vi "DSF.Engine.Interface.RT FIFO.Create.vi"(7 "size (10)":u32, 8 "error in (no error)":errorcluster) -> (0 "error out":errorcluster, 3 "RT FIFO":T1)   [LabVIEW 2016, in "DSF.Engine.lvlib" / "DSF.Engine.Interface.lvclass"]
uses:
  DSF.Engine.Interface.lvclass
  DSF.Engine.Interface.RT FIFO Ref.ctl
  DSF.Engine.Interface.RT FIFO Data.ctl
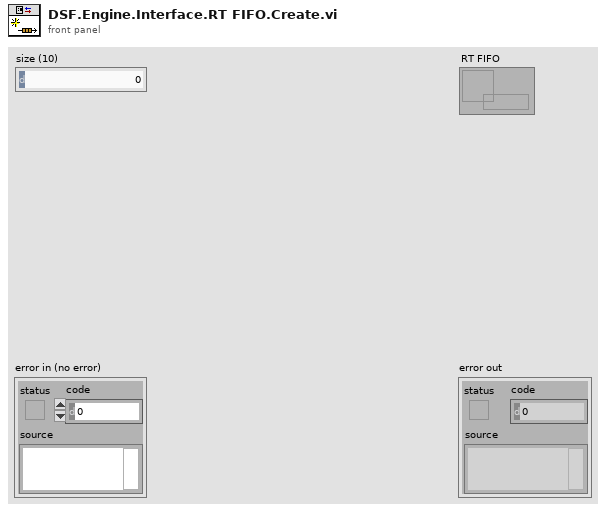
[diagram p1: front panel]
types:
  T1 = typedef "DSF.Engine.lvlib/DSF.Engine.Interface.lvclass/DSF.Engine.Interface.RT FIFO Ref.ctl" = refnum<k33>
  T2 = typedef "DSF.Engine.lvlib/DSF.Engine.Interface.lvclass/DSF.Engine.Interface.RT FIFO Data.ctl" = cluster{"Command":u8, "Payload":u64}
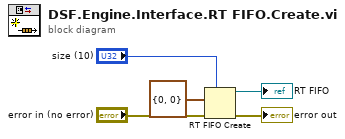
[diagram p0: block diagram]
diagram:
  n1 = RT FIFO Create(1:T2 {"Command"=0, "Payload"=0} ("Cluster"), 3:"error in (no error)", 4:"size (10)") -> (8:→"RT FIFO":refnum<k33>, 11:→"error out":errorcluster)  [unwired: 5 in, 1 out]
